vi "replace_controls.vi"(8 "error in (no error)":errorcluster, 10 "Path to new control":path, 11 "VI in":refnum<vi>) -> (0 "error out":errorcluster, 3 "VI out":refnum<vi>)   [LabVIEW 2020]
uses:
  <vilib>/Utility/traverseref.llb/TRef TravTarget.ctl
  <vilib>/Utility/traverseref.llb/VI Scripting - Traverse.lvlib
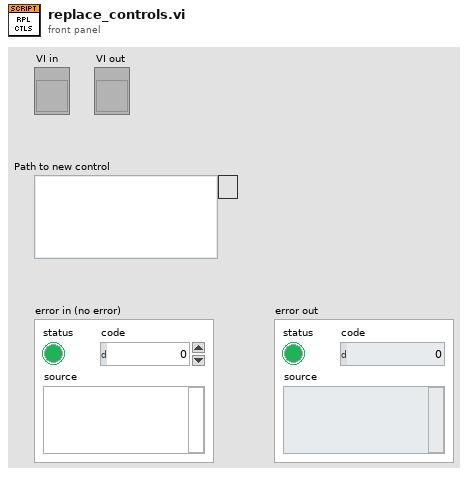
[diagram p1: front panel]
types:
  T1 = typedef "TRef TravTarget.ctl" = enum16{"FP", "BD", "Other"}
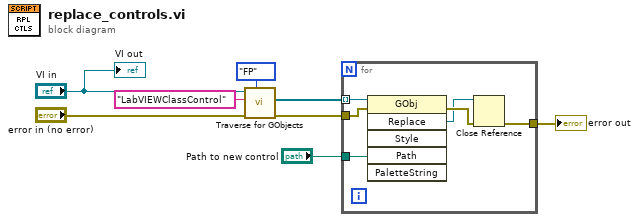
[diagram p0: block diagram]
diagram:
  n1 = call <vilib>:"Traverse for GObjects.vi"("Traverse Target"=TRef_TravTarget."FP", "error in (no error)"="error in (no error)", "Class Name"="LabVIEWClassControl", "VI Refnum"="VI in") -> ("error out"=w6:errorcluster, "References"=w3:refnum<vi>[])  [unwired: 4 in, 2 out]
  n2 = for {
    tunnel: w3 -> [w14] mode=indexing
    tunnel: "Path to new control" -> [w13]
    tunnel: w6 -> [w12]
    tunnel: [w9] -> w8
    n3 = invoke class="GObj" method="Replace"(reference=w14, error in=w12, "Path"=w13) -> (error out=w11:errorcluster, "Replace"=w10:refnum<vi>)  [unwired: 3 in, 4 out]
    n4 = Close Reference(reference=w10, error in (no error)=w11) -> (error out=w9:errorcluster)
  }
  "error out" <- w8
  "VI out" <- "VI in"
